vi "1_3.vi"() -> ()   [LabVIEW 2019]
doc: "Demonstrates the use of the Sample Compression Express VI."
panel:
  in  "stop":bool
  out "Sine":dynamicdata(graph)
  in  "Enable":bool=TRUE
  out "Mean":dbl
  # "Overview: Demonstrates the use of the Sample Compression Express VI.\nInstructions:\n1. Run the VI.\n2. The Sine with Noise plot contains 100 samples.\n3. The Sine with Noise (Max) plot is the result of Sample Compression, configured with a reduction factor of 10 and a reduction method of Maximum.\n4. Open the block diagram. Right-click on the Sample Compression Express VI and select Properties from the menu.\n5. Experiment with the other configuration options for the Sample Compression Express VI."
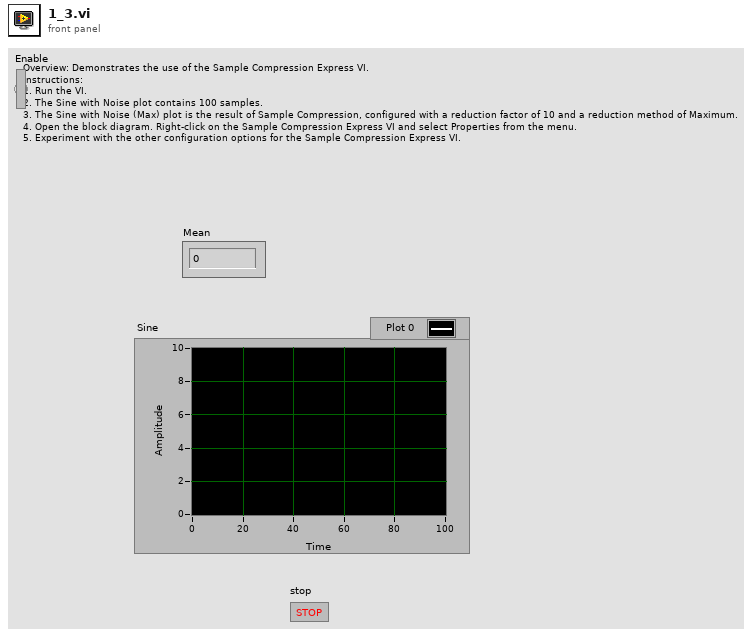
[diagram p1: front panel]
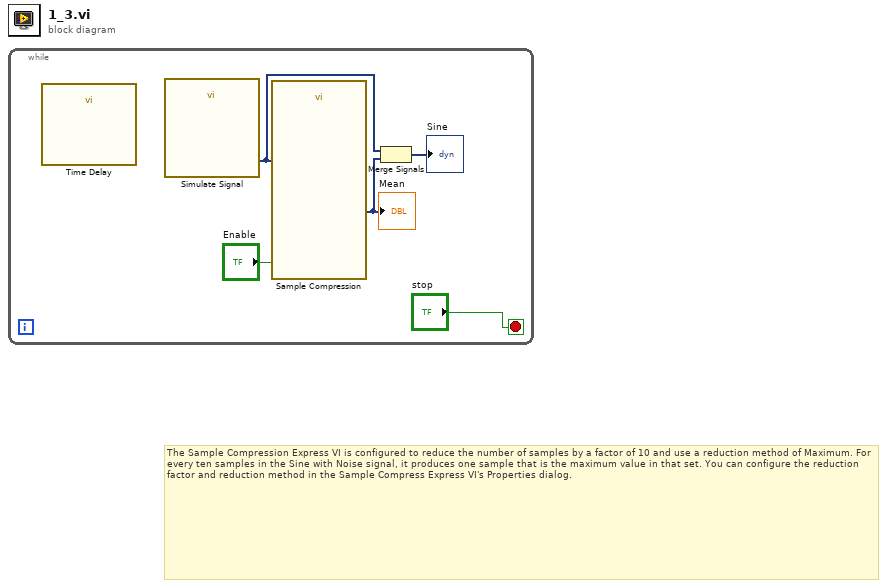
[diagram p0: block diagram]
diagram:
  # "The Sample Compression Express VI is configured to reduce the number of samples by a factor of 10 and use a reduction method of Maximum. For every ten samples in the Sine with Noise signal, it produces one sample that is the maximum value in that set. You can configure the reduction factor and reduction method in the Sample Compress Express VI's Properties dialog."
  n1 = while {
    stop <- "stop" stop-if-true
    n2 = call "Time Delay"() -> ()  [unwired: 11 in, 1 out]
    n3 = call "Simulate Signal"() -> ("Sine"=w5:dynamicdata)  [unwired: 14 in, 1 out]
    n4 = call "Sample Compression"("Enable"="Enable", "Signals"=w5) -> ("Mean"=w3:dynamicdata)  [unwired: 7 in, 2 out]
    "Mean" <- w3
    n5 = Merge Signals(w5, w3) -> (→"Sine":dynamicdata)
  }
